vi "How Read_Write Binary file output.vi"() -> ()   [LabVIEW 2020]
panel:
  out "Waveform Graph":dbl[](graph)
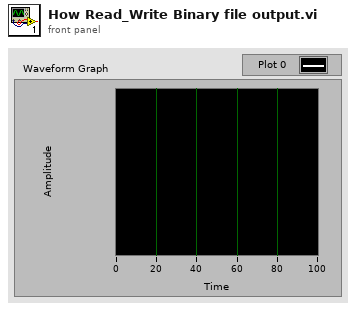
[diagram p1: front panel]
types:
  T1 = enum16{"open", "replace", "create", "open or create", "replace or create", "replace or create with confirmation"}
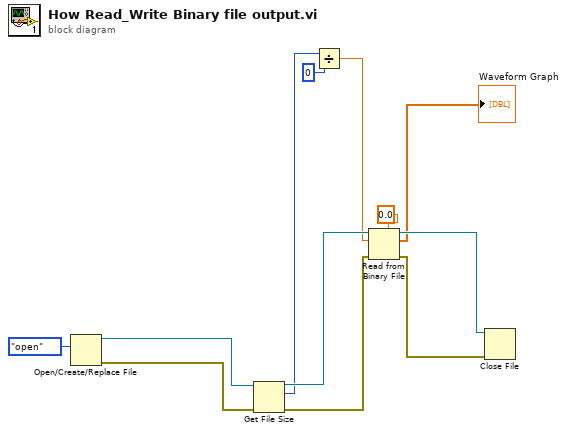
[diagram p0: block diagram]
diagram:
  n1 = Open/Create/Replace File(operation (0:open)=T1."open") -> (refnum out=w8:refnum<file>, error out=w7:errorcluster)  [unwired: 5 in, 1 out]
  n2 = Get File Size(file=w8, error in=w7) -> (refnum out=w5:refnum<file>, size (in bytes)=w4:i64, 0:w6:errorcluster)
  n3 = Divide(x=w4, y=0) -> (x/y=w2:dbl)
  n4 = Read from Binary File(5:0.0, 8:w6, 10:w2, 11:w5) -> (0:w10:errorcluster, 2:→"Waveform Graph":dbl[], 3:w11:refnum<file>)  [unwired: 2 in, 1 out]
  n5 = Close File(refnum=w11, error in=w10) -> ()  [unwired: 2 out]
